vi "Laser Turret 2.vi"() -> ()   [LabVIEW 2022 SP3]
uses:
  <vilib>/userdefined/High Color/IMAQdx.ctl
  <vilib>/MakerHub/LINX/Public/Peripherals/Digital/Digital Write 1 Chan.vi
  <vilib>/MakerHub/LINX/Public/Peripherals/Digital/Digital Write N Chans.vi
  <vilib>/MakerHub/LINX/Private/Local IO/LinxDigitalWrite.vi
  <vilib>/MakerHub/LINX/Public/Utilities/Check Channel.vi
  <vilib>/MakerHub/LINX/Public/Utilities/Open Serial.vi
  <vilib>/MakerHub/LINX/Public/Sensors/Motion/Servo/Servo Open N Channels.vi
  <vilib>/MakerHub/LINX/Private/Utilties/Generate Error.vi
  <vilib>/MakerHub/LINX/Public/Sensors/Motion/Servo/Servo Set Pulse Width N Channels.vi
  <vilib>/MakerHub/LINX/Public/Sensors/Motion/Servo/Servo Close N Channels.vi
  <vilib>/MakerHub/LINX/LMH-LINX.lvlib
  <vilib>/MakerHub/LINX/Public/Sensors/Motion/Servo/Servo.lvlib
  <vilib>/vision/driver/NI_Vision_Acquisition_Software.lvlib
panel:
  in  "stop":bool
  in  "Laser Channel":u8
  in  "Laser":bool
  in  "Camera":T1
  out "Turret Vision":T2(plugin-control)
  out "Mouse Control":picture
  in  "Left-Right":u16(slide)=2200 step=100 scale=500.0..2500.0
  in  "Up-Down":u16(slide)=1400 step=100 scale=500.0..2500.0
  in  "Servo Channels":u8[](array[numeric])
  out "Device Name":string
  in  "Stop":bool
  # "Setup"
  # "Main Controls"
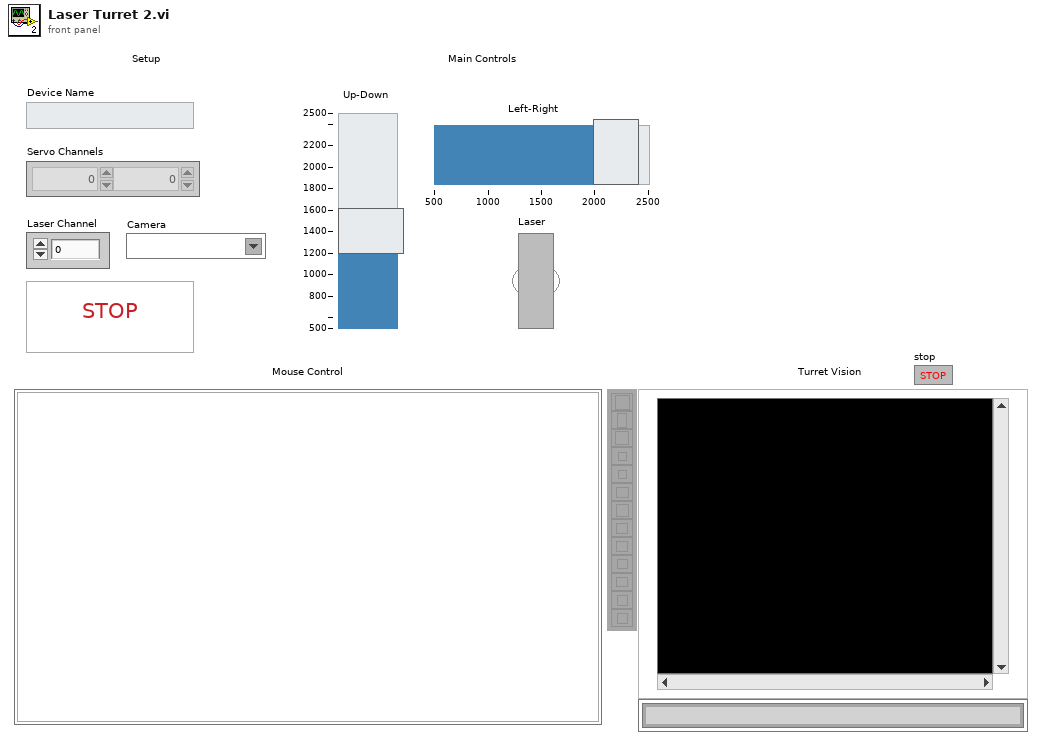
[diagram p1: front panel]
types:
  T1 = typedef "IMAQdx.ctl" = refnum<k21>
  T2 = typedef "IMAQ Image.ctl" = refnum<image>
  T3 = typedef "LMH-LINX.lvlib/LINX Ref.ctl" = cluster{"IO":T4, "Interface":T5, "LINX Device Config":T6}
  T4 = typedef "LMH-LINX.lvlib/Platform.ctl" = enum16{"Remote", "Local"}
  T5 = typedef "LMH-LINX.lvlib/Interface.ctl" = enum16{"Serial", "TCP"}
  T6 = typedef "LMH-LINX.lvlib/Device.lvlib/LINX Device Config.ctl" = cluster{"Interface":T5, "COM Port":refnum<visa-resource-name>, "TCP Configuration":T7, "Device Family":u8, "Device ID":u8, "Device Name":string, "TCP Ref":refnum<k5>, "Channels":T8}
  T7 = typedef "LMH-LINX.lvlib/Device.lvlib/TCP Config.ctl" = cluster{"IP Address":string, "Port":u16}
  T8 = typedef "LMH-LINX.lvlib/Channels.ctl" = cluster{"DI":u8[], "DO":u8[], "AI":u8[], "AO":u8[], "PWM":u8[], "QE":u8[], "UART":u8[], "I2C 2":u8[], "SPI":u8[], "CAN":u8[], "Servo":u8[], "AI Ref (V)":dbl, "AI Resolution (Bits)":u8, "AO Ref (V)":dbl, "AO Resolution (Bits)":u8}
  T9 = typedef "eventvkey.ctl" = enum16{"ASCII", "Enter", "Return", "Shift", "Ctrl", "Alt", "Cmd", "Opt", "Caps", "NumLock", "Clear", "Break", "Up", "Down", "Left", "Right", "Insert", "Delete", "Home", "End", "PageUp", "PageDown", "Escape", "Help", "Pause", "ScrollLock", "F1", "F2", "F3", "F4", "F5", "F6", "F7", "F8", "F9", "F10", "F11", "F12", "F13", "F14", "F15", "F16", "F17", "F18", "F19", "F20", "F21", "F22", "F23", "F24", "Play", "VolumeUp", "VolumeDown", "Mute", "Two Byte Char"}
  T10 = typedef "LVMouseTypeDef.ctl" = cluster{"Mouse Position":cluster{"X":i32, "Y":i32}, "Mouse Modifiers":cluster{"Button Down":bool, "Shift Mod":bool, "Menu Mod":bool, "Option Mod":bool}}
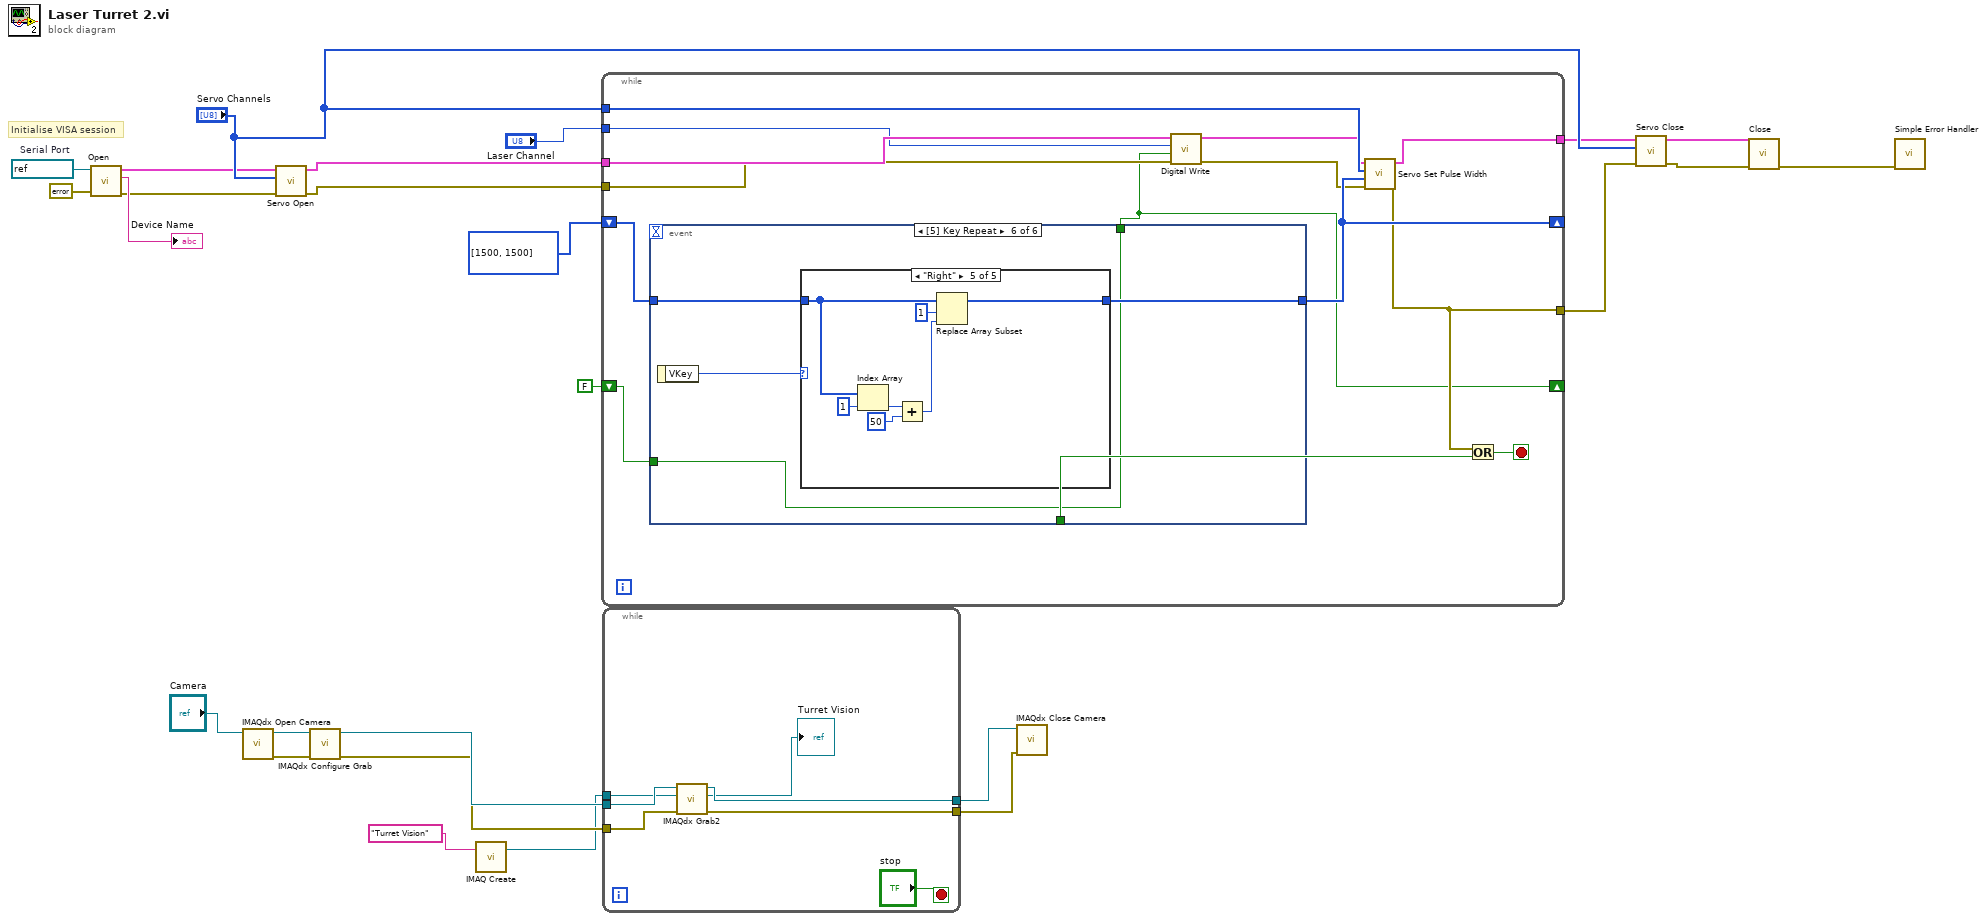
[diagram p0: block diagram]
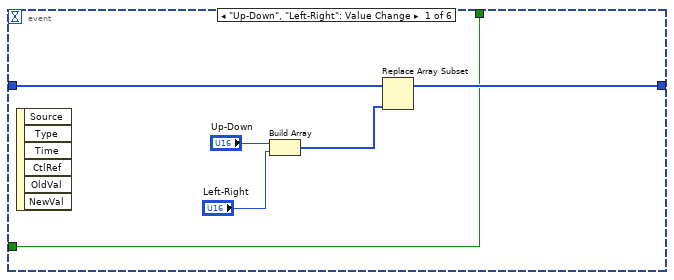
[diagram p2: hidden frame]
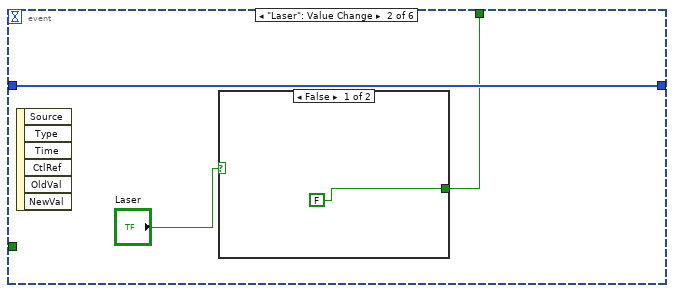
[diagram p3: hidden frame]
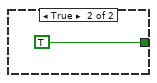
[diagram p4: hidden frame]
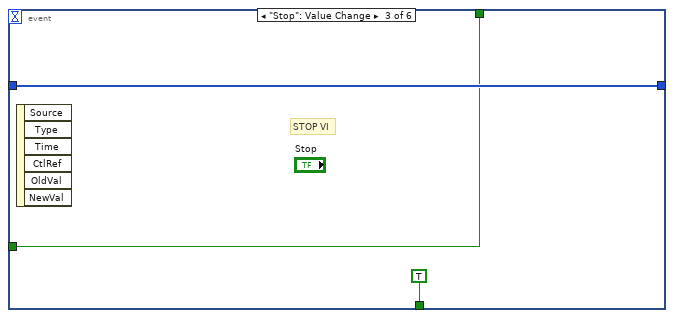
[diagram p5: hidden frame]
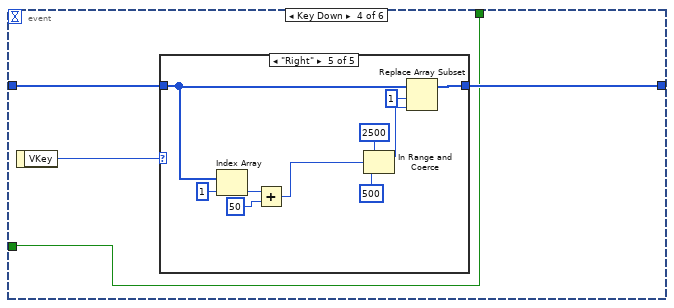
[diagram p6: hidden frame]
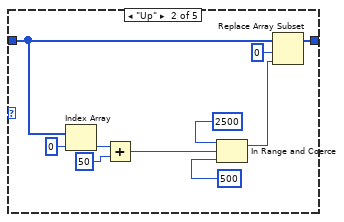
[diagram p8: hidden frame]
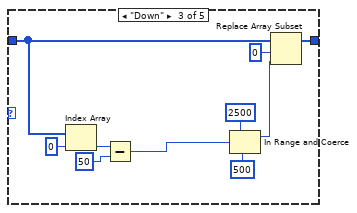
[diagram p9: hidden frame]
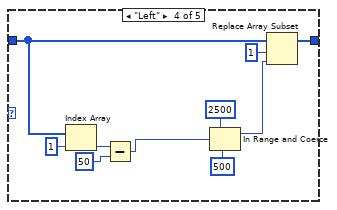
[diagram p10: hidden frame]
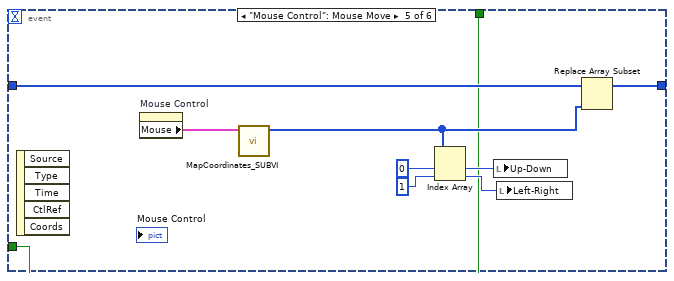
[diagram p11: hidden frame]
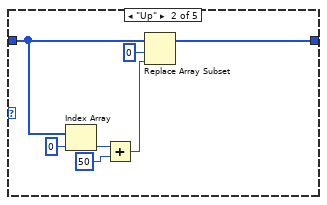
[diagram p13: hidden frame]
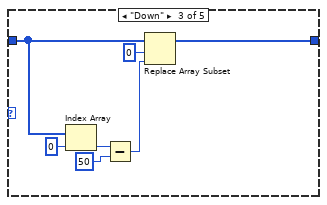
[diagram p14: hidden frame]
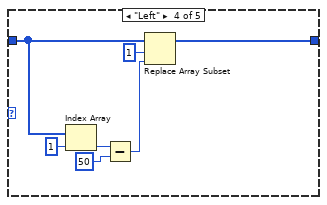
[diagram p15: hidden frame]
diagram:
  w25 = refnum<visa-resource-name> "COM5"  # Serial Port
  # "Initialise VISA session"
  n1 = call-poly <vilib>:"Open.vi"("Error In"=errorcluster {"status"=FALSE, "code"=0, "source"=""}, "Serial Port"=w25) -> ("Error Out"=w19:errorcluster, "Device Name"=→"Device Name":string, "LINX Resource"=w5:T3)  [unwired: 7 in]
  n2 = call <vilib>:"IMAQdx Open Camera.vi"("Session In"="Camera") -> ("error out"=w14:errorcluster, "Session Out"=w13:T1)  [unwired: 9 in]
  n3 = call-poly <vilib>:"Servo Open.vi"("Error In"=w19, "Servo Channels"="Servo Channels", "LINX Resource"=w5) -> ("Error Out"=w18:errorcluster, "LINX Resource"=w20:T3)  [unwired: 7 in]
  n4 = call <vilib>:"IMAQdx Configure Grab.vi"("error in"=w14, "Session In"=w13) -> ("error out"=w11:errorcluster, "Session Out"=w12:T1)  [unwired: 8 in]
  n5 = call "IMAQ Create"("Image Name"="Turret Vision") -> ("New Image"=w8:T2)  [unwired: 4 in, 1 out]
  n6 = while {
    tunnel: w20 -> [w33]
    tunnel: w18 -> [w32]
    tunnel: "Servo Channels" -> [w37]
    shift-right: [w36] -> _
    shift-left: u16[] [1500, 1500] -> [w38]
    tunnel: [w35] -> w17
    tunnel: [w34] -> w4
    tunnel: "Laser Channel" -> [w29]
    shift-right: [w27] -> _
    shift-left: FALSE -> [w28]
    stop <- w26 stop-if-true
    n7 = event shown="[5] Key Repeat" {
      selector: _ -> [_ _ _ _ _ _]
      dyn-events: _ -> [_ _ _ _ _ _]
      timeout: _ -> [_ _ _ _ _ _]
      tunnel: [_ _ TRUE ("Stop") _ _ _] -> w39
      tunnel: [w42 w48 w52 w55 w106 w109] -> w36
      tunnel: w38 -> [w43 w48 w52 w56 w105 w110]
      tunnel: [w40 w47 w51 w54 w99 w108] -> w27
      tunnel: w28 -> [w40 _ w51 w54 w99 w108]
      event "Up-Down", "Left-Right": Value Change {
        n8 = event-data() -> ()  [unwired: 1 in, 6 out]
        n9 = Build Array("Up-Down", "Left-Right") -> (w41:u16[])
        n10 = Replace Array Subset(array=w43, new element=w41) -> (w42:u16[])  [unwired: 1 in]
      }
      event "Laser": Value Change {
        n11 = event-data() -> ()  [unwired: 1 in, 6 out]
        n12 = case shown="False" "Laser" {
          tunnel: [FALSE TRUE] -> w47
          frame False {
          }
          frame True {
          }
        }
      }
      event "Stop": Value Change {
        # "STOP VI"
        n13 = event-data() -> ()  [unwired: 1 in, 6 out]
      }
      event Key Down {
        n14 = event-data() -> ("VKey"=w57:T9)  [unwired: 1 in]
        n15 = case shown="\"Right\"" w57 {
          tunnel: w56 -> [w58 w66 w76 w86 w96]
          tunnel: [w58 w68 w78 w88 w98] -> w55
          frame "ASCII", Default {
            # "do nothing"
          }
          frame "Up" {
            n16 = Index Array(array=w66, index=0) -> (element=w64:u16)
            n17 = Add(x=w64, y=u16 50) -> (x+y=w62:u16)
            n18 = In Range and Coerce(upper limit=u16 2500, x=w62, lower limit=u16 500 ("x+y")) -> (coerced(x)=w60:u16)  [unwired: 1 out]
            n19 = Replace Array Subset(array=w66, new element=w60, index=0) -> (w68:u16[])
          }
          frame "Down" {
            n20 = Index Array(array=w76, index=0) -> (element=w74:u16)
            n21 = Subtract(x=w74, y=u16 50) -> (x-y=w70:u16)
            n22 = In Range and Coerce(upper limit=u16 2500, x=w70, lower limit=u16 500 ("x+y")) -> (coerced(x)=w69:u16)  [unwired: 1 out]
            n23 = Replace Array Subset(array=w76, new element=w69, index=0) -> (w78:u16[])
          }
          frame "Left" {
            n24 = Index Array(array=w86, index=1) -> (element=w84:u16)
            n25 = Subtract(x=w84, y=u16 50) -> (x-y=w79:u16)
            n26 = In Range and Coerce(upper limit=u16 2500, x=w79, lower limit=u16 500 ("x+y")) -> (coerced(x)=w82:u16)  [unwired: 1 out]
            n27 = Replace Array Subset(array=w86, new element=w82, index=1) -> (w88:u16[])
          }
          frame "Right" {
            n28 = Index Array(array=w96, index=1) -> (element=w94:u16)
            n29 = Add(x=w94, y=u16 50) -> (x+y=w90:u16)
            n30 = In Range and Coerce(upper limit=u16 2500, x=w90, lower limit=u16 500 ("x+y")) -> (coerced(x)=w89:u16)  [unwired: 1 out]
            n31 = Replace Array Subset(array=w96, new element=w89, index=1) -> (w98:u16[])
          }
        }
      }
      event "Mouse Control": Mouse Move {
        n32 = event-data() -> ()  [unwired: 1 in, 5 out]
        n33 = property on="Mouse Control" class="Pict"() -> ("Mouse"=w107:T10)  [unwired: 2 in, 2 out]
        n34 = call "MapCoordinates_SUBVI.vi"("Mouse"=w107) -> ("Pulse Width Array"=w104:u16[])  [unwired: 10 in]
        n35 = Index Array(array=w104, index #1=0 ("index"), index #2=1 ("index")) -> (element #1=w100:u16, element #2=w101:u16)
        n36 = local write "Up-Down"(w100) -> ()
        n37 = local write "Left-Right"(w101) -> ()
        n38 = Replace Array Subset(array=w105, new element=w104) -> (w106:u16[])  [unwired: 1 in]
      }
      event Key Repeat {
        n39 = event-data() -> ("VKey"=w111:T9)  [unwired: 1 in]
        n40 = case shown="\"Right\"" w111 {
          tunnel: w110 -> [w112 w117 w124 w131 w138]
          tunnel: [w112 w119 w126 w133 w140] -> w109
          frame "ASCII", Default {
            # "do nothing"
          }
          frame "Up" {
            n41 = Index Array(array=w117, index=0) -> (element=w115:u16)
            n42 = Add(x=w115, y=u16 50) -> (x+y=w113:u16)
            n43 = Replace Array Subset(array=w117, new element=w113, index=0) -> (w119:u16[])
          }
          frame "Down" {
            n44 = Index Array(array=w124, index=0) -> (element=w122:u16)
            n45 = Subtract(x=w122, y=u16 50) -> (x-y=w120:u16)
            n46 = Replace Array Subset(array=w124, new element=w120, index=0) -> (w126:u16[])
          }
          frame "Left" {
            n47 = Index Array(array=w131, index=1) -> (element=w129:u16)
            n48 = Subtract(x=w129, y=u16 50) -> (x-y=w127:u16)
            n49 = Replace Array Subset(array=w131, new element=w127, index=1) -> (w133:u16[])
          }
          frame "Right" {
            n50 = Index Array(array=w138, index=1) -> (element=w136:u16)
            n51 = Add(x=w136, y=u16 50) -> (x+y=w134:u16)
            n52 = Replace Array Subset(array=w138, new element=w134, index=1) -> (w140:u16[])
          }
        }
      }
    }
    n53 = call-poly <vilib>:"Digital Write.vi"("Error In"=w32, "Output Value"=w27, "DO Channel"=w29, "LINX Resource"=w33) -> ("Error Out"=w30:errorcluster, "LINX Resource"=w31:T3)  [unwired: 6 in]
    n54 = call-poly <vilib>:"Servo Set Pulse Width.vi"("Error In"=w30, "Pulse Widths (uS)"=w36, "Servo Channels"=w37, "LINX Resource"=w31) -> ("Error Out"=w35:errorcluster, "LINX Resource"=w34:T3)  [unwired: 6 in]
    n55 = Or(x=w35, y=w39) -> (x .or. y?=w26:bool)
  }
  n56 = while {
    tunnel: w12 -> [w147]
    tunnel: w11 -> [w146]
    tunnel: [w145] -> w10
    tunnel: [w144] -> w9
    tunnel: w8 -> [w143]
    stop <- "stop" stop-if-true
    n57 = call <vilib>:"IMAQdx Grab2.vi"("error in"=w146, "Image In"=w143, "Session In"=w147) -> ("error out"=w144:errorcluster, "Image Out"=→"Turret Vision":T2, "Session Out"=w145:T1)  [unwired: 5 in, 1 out]
  }
  n58 = call <vilib>:"IMAQdx Close Camera.vi"("error in"=w9, "Session In"=w10) -> ()  [unwired: 9 in, 1 out]
  n59 = call-poly <vilib>:"Servo Close.vi"("Error In"=w17, "Servo Channels"="Servo Channels", "LINX Resource"=w4) -> ("Error Out"=w21:errorcluster, "LINX Resource"=w3:T3)  [unwired: 7 in]
  n60 = call <vilib>:"Close.vi"("Error In"=w21, "LINX Resource"=w3) -> ("Error Out"=w22:errorcluster)  [unwired: 9 in]
  n61 = call <vilib>:"Simple Error Handler.vi"("error in (no error)"=w22) -> ()  [unwired: 4 in, 5 out]
